vi "report.vi"(5 "Rname":string, 7 "date":string, 8 "error in (no error)":errorcluster, 9 "pruefer":string, 10 "obnr":string, 11 "Report in":refnum<class "Report.lvclass">) -> (0 "error out":errorcluster, 3 "Report out":refnum<class "Report.lvclass">)   [LabVIEW 2013, in "DatenKlassen.lvlib" / "Report.lvclass"]
doc: "Konstruktor für das Report Objekt"
uses:
  Report.lvclass
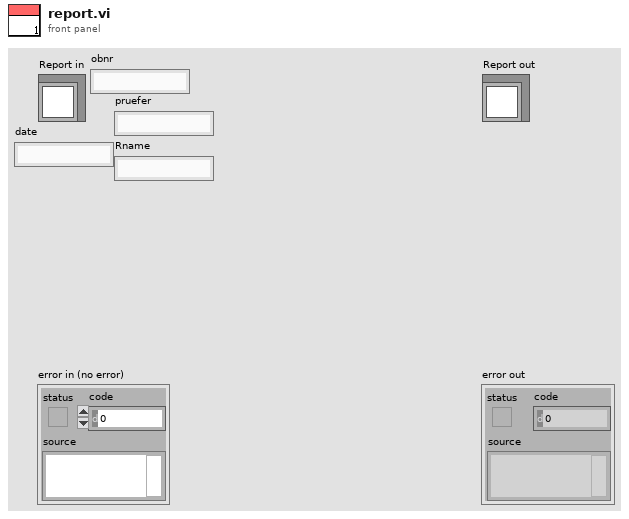
[diagram p1: front panel]
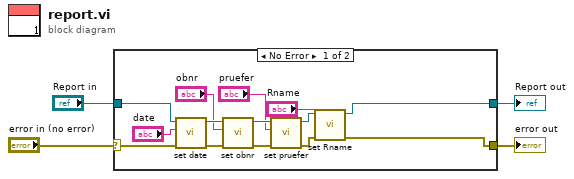
[diagram p0: block diagram]
diagram:
  n1 = case shown="No Error" "error in (no error)" {
    selector: "error in (no error)" -> [w13 w20]
    tunnel: [w5 w20] -> w3
    tunnel: [w6 w19] -> w1
    tunnel: "Report in" -> [w16 w19]
    frame No Error {
      n2 = call-dynamic "set date.vi"("error in (no error)"=w13, "date"="date", "Report (Eingang)"=w16) -> ("error out"=w15:errorcluster, "Report (Ausgang)"=w18:refnum<class "Report.lvclass">)  [unwired: 7 in]
      n3 = call-dynamic "set obnr.vi"("error in (no error)"=w15, "obnr"="obnr", "Report in"=w18) -> ("error out"=w14:errorcluster, "Report out"=w17:refnum<class "Report.lvclass">)  [unwired: 7 in]
      n4 = call-dynamic "set pruefer.vi"("error in (no error)"=w14, "pruefer"="pruefer", "Report in"=w17) -> ("error out"=w9:errorcluster, "Report out"=w8:refnum<class "Report.lvclass">)  [unwired: 7 in]
      n5 = call-dynamic "set Rname.vi"("error in (no error)"=w9, "Rname"="Rname", "Report (Eingang)"=w8) -> ("error out"=w5:errorcluster, "Report (Ausgang)"=w6:refnum<class "Report.lvclass">)  [unwired: 7 in]
    }
    frame Error {
    }
  }
  "error out" <- w3
  "Report out" <- w1
